vi "Ask for Run Config.vi"(8 "error in (no error)":errorcluster, 11 "Guardian in":refnum<class "Guardian.lvclass">) -> (0 "error out":errorcluster, 3 "Guardian out":refnum<class "Guardian.lvclass">)   [LabVIEW 2026, in "TALOS.lvlib" / "Guardian.lvlib" / "Guardian.lvclass"]
uses:
  Guardian.lvclass
  C:/LabVIEW Code/TALOS/talos/Ancestor/Ancestor/Ancestor.lvclass
  C:/LabVIEW Code/TALOS/builds/Actor Framework PPL/Actor Framework.lvlibp/1abvi3w/vi.lib/ActorFramework/Actor/Actor.lvclass
  Ancestor/Ancestor/Infinite Message Selector.ctl
  Ancestor/Ancestor/Ancestor.lvclass/Ancestor.ctl
  Guardian Messages/Message to uService Msg/Message to uService Msg.lvclass/Message to uService Msg.ctl
  Ancestor/Ancestor/Read ID.vi
  builds/Actor Framework PPL/Actor Framework.lvlibp/1abvi3w/vi.lib/ActorFramework/Message Enqueuer/Enqueue.vi
  Guardian Messages/Message to uService Msg/Message to uService Msg.lvclass
  builds/Actor Framework PPL/Actor Framework.lvlibp/1abvi3w/vi.lib/ActorFramework/Actor/Actor.lvclass
  Ancestor/Ancestor/Ancestor.lvclass
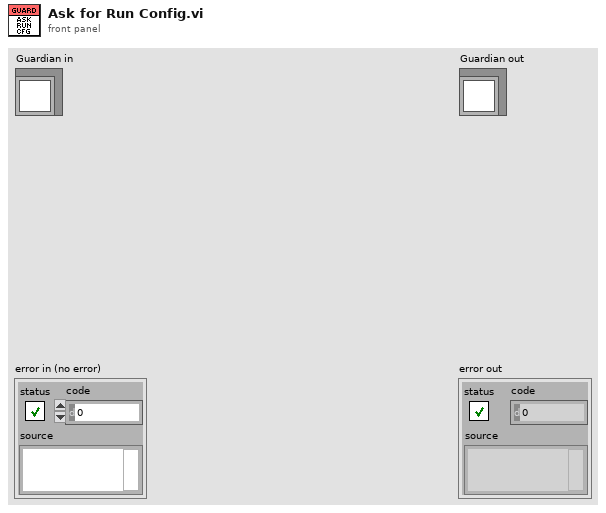
[diagram p1: front panel]
types:
  T1 = typedef "TALOS.lvlib/Ancestor.lvlib/Ancestor.lvclass/Infinite Message Selector.ctl" = enum16{"Start", "Stop", "Check", "Flush (Stop all)", "Init"}
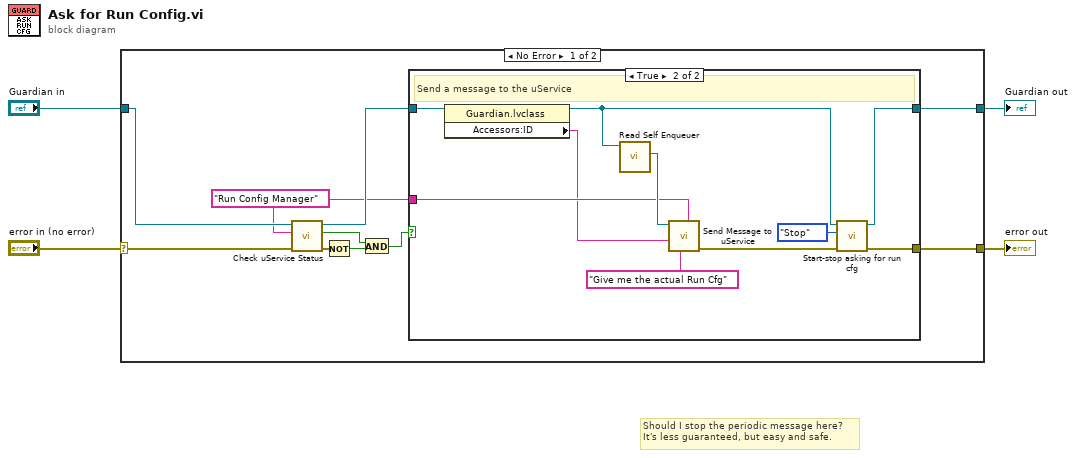
[diagram p0: block diagram]
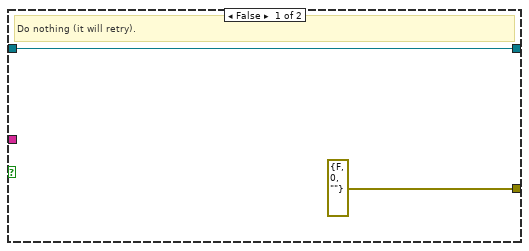
[diagram p2: hidden frame]
diagram:
  # "Should I stop the periodic message here?\nIt's less guaranteed, but easy and safe."
  n1 = case shown="No Error" "error in (no error)" {
    selector: "error in (no error)" -> [w13 w28]
    tunnel: [w11 w28] -> w3
    tunnel: [w10 w27] -> w1
    tunnel: "Guardian in" -> [w14 w27]
    frame No Error {
      w9 = "Run Config Manager" ("uService ID")
      n2 = call-dynamic "Check uService Status.vi"("error in (no error)"=w13, "uService ID"=w9, "Ancestor in"=w14) -> ("error out"=w5:errorcluster, "Online?"=w8:bool, "Ancestor out"=w12:refnum<class "Guardian.lvclass">)  [unwired: 5 in, 1 out]
      n3 = Not(x=w5) -> (.not. x?=w6:bool)
      n4 = And(x=w8, y=w6) -> (x .and. y?=w7:bool)
      n5 = case shown="True" w7 {
        tunnel: w12 -> [w16 w20]
        tunnel: [errorcluster {"status"=FALSE, "code"=0, "source"=""} ("error out") w22] -> w11
        tunnel: [w16 w21] -> w10
        tunnel: w9 -> [_ w25]
        frame False {
          # "Do nothing (it will retry)."
        }
        frame True {
          # "Send a message to the uService"
          n6 = property class="Guardian.lvclass"(reference=w20) -> (reference out=w18:refnum<class "Guardian.lvclass">, "Accessors:ID"=w17:string)  [unwired: 1 in, 1 out]
          n7 = call "Read Self Enqueuer.vi"("Actor"=w18) -> ("Self Enqueuer"=w26:refnum<class "Message Enqueuer.lvclass">)  [unwired: 10 in]
          n8 = call "Send Message to uService.vi"("uService ID"=w25, "Message"="Give me the actual Run Cfg", "Data"=w17, "Message Enqueuer"=w26) -> ("error out"=w23:errorcluster)  [unwired: 6 in, 1 out]
          n9 = call-dynamic "Start-stop asking for run cfg.vi"("error in (no error)"=w23, "Infinite Message Selector"=Infinite_Message_Selector."Stop", "Guardian in"=w18) -> ("error out"=w22:errorcluster, "Guardian out"=w21:refnum<class "Guardian.lvclass">)  [unwired: 7 in]
        }
      }
    }
    frame Error {
    }
  }
  "error out" <- w3
  "Guardian out" <- w1
